vi "NormalizeAngle.vi"(1 "angle (rad)":dbl) -> (0 "angle (between pi and -pi)":dbl(knob) scale=3.14159..-3.14159)   [LabVIEW 2016, in "Team900SwerveDrive.lvlib"]
uses:
  Team900SwerveDrive.lvlib
panel:
  # "This takes an angle of any finite value and\noutputs the same angle between pi and -pi"
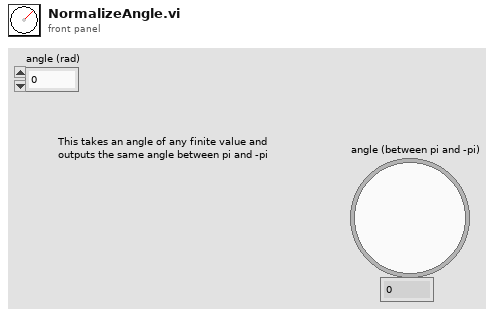
[diagram p1: front panel]
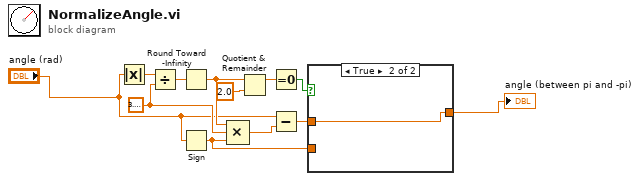
[diagram p0: block diagram]
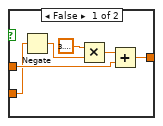
[diagram p2: hidden frame]
diagram:
  w9 = 3.141592653589793
  n1 = Absolute Value(x="angle (rad)") -> (abs(x)=w12:dbl)
  n2 = Divide(x=w12, y=w9) -> (x/y=w11:dbl)
  n3 = Round Toward -Infinity(1:w11) -> (0:w8:dbl)
  n4 = Sign(1:"angle (rad)") -> (0:w3:dbl)
  n5 = Compound Arithmetic op=MULTIPLY(w8, w9, w3) -> (w10:dbl)
  n6 = Quotient & Remainder(x=w8, y=2.0) -> (x-y*floor(x/y)=w6:dbl)  [unwired: 1 out]
  n7 = Equal To 0?(x=w6) -> (x = 0?=w4:bool)
  n8 = Subtract(x="angle (rad)", y=w10) -> (x-y=w5:dbl)
  n9 = case shown="True" w4 {
    tunnel: [w17 w19] -> w1
    tunnel: w5 -> [w18 w19]
    tunnel: w3 -> [w16 _]
    frame False {
      n10 = Negate(x=w16) -> (-x=w14:dbl)
      n11 = Multiply(x=3.141592653589793, y=w14) -> (x*y=w13:dbl)
      n12 = Add(x=w13, y=w18) -> (x+y=w17:dbl)
    }
    frame True {
    }
  }
  "angle (between pi and -pi)" <- w1
